vi "ADV_and_HF.vi"() -> (5 "Plug in titles":string[](array[string]), 7 "Plug in values":string[](array[string]))   [LabVIEW 2010]
uses:
  Controls/Post_Process.ctl
  Globals/Meas_global.vi
  Globals/Plug_in_data_global.vi
  <vilib>/Analysis/NI_AALBase.lvlib
panel:
  in  "Case Constant\n(See Context Help)":bool=TRUE
  out "Hot Film mean":dbl format="%.2f"
  out "ADV mean":dbl format="%.2f"
  in  "Approx period":dbl=38.0 format="%.2f"
  in  "End chop":i32
  in  "Start chop":i32
  out "Auto End Chop":i32
  out "Product":dbl[][](graph)
  out "Hot Film":dbl[][](graph)
  out "ADV":dbl[][](graph)
  out "Hot Film Auto correlation":cluster{dbl, dbl, dbl[]}(graph)
  out "ADV Auto correlation":cluster{dbl, dbl, dbl[]}[](graph)
  out "Correlation Coefficient":T1(graph)
  out "Clipped length":i32
  out "Auto Start Chop":i32
  out "V components":cluster{dbl[], dbl[]}[](graph)
  out "U components":cluster{dbl[], dbl[]}[](graph)
  # "End chop"
  # "End chop"
  # "Amount Hot Film leads ADV"
  # "End chop"
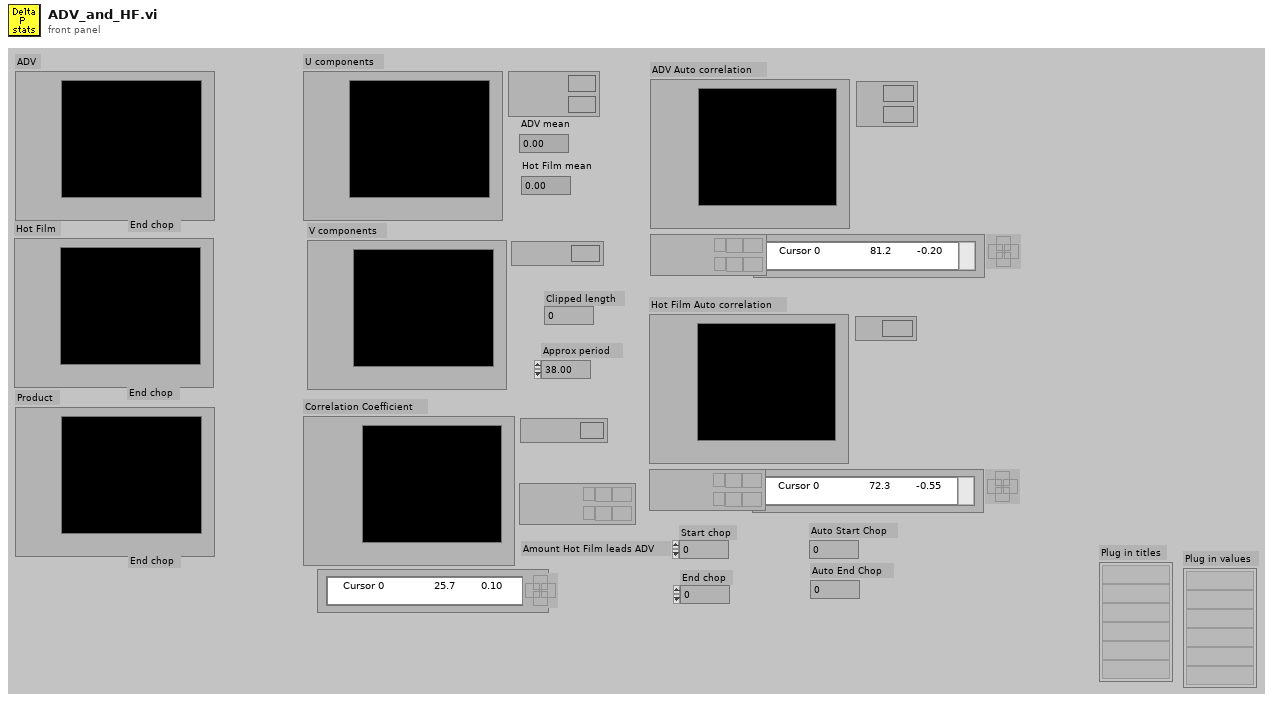
[diagram p1: front panel]
types:
  T1 = cluster{"Time":dbl[], "Correlation Coefficient":dbl[]}
  T2 = typedef "Post_Process.ctl" = enum16{"Take New Data", "Post Process Raw Data File"}
  T3 = typedef "Analysis_info_cluster.ctl" = cluster{"Colour":u32, "Inst type":T4, "Inst name":string, "Symbol":string, "Code name":string, "Extra Info":string, "Inst Array":T5, "Index":i32, "Voltage Index":i32, "Extra Titles":string[], "Extra Values":string[]}
  T4 = typedef "Inst_type.ctl" = enum16{"Propeller anemometer", "Raw voltage", "Pressure Transducer", "Pitot-static tube", "Preston tube", "Hot wire", "Cross wire 1", "Cross wire 2", "Generic Linear", "Generic Polynomial", "Generic BackPoly", "Fast FID", "Thermocouple", "Cold wire", "Pulsed Wire", "LDA Vel", "LDA Tran time", "LDA Arr time"}
  T5 = typedef "Instrument_Array.ctl" = enum16{"PWA", "LDA", "Analogue"}
  T6 = cluster{"Name":string, "X":dbl, "Y":dbl, "Z":dbl}[]
  T7 = cluster{"Name":string, "X":dbl, "Y":dbl, "Z":dbl}
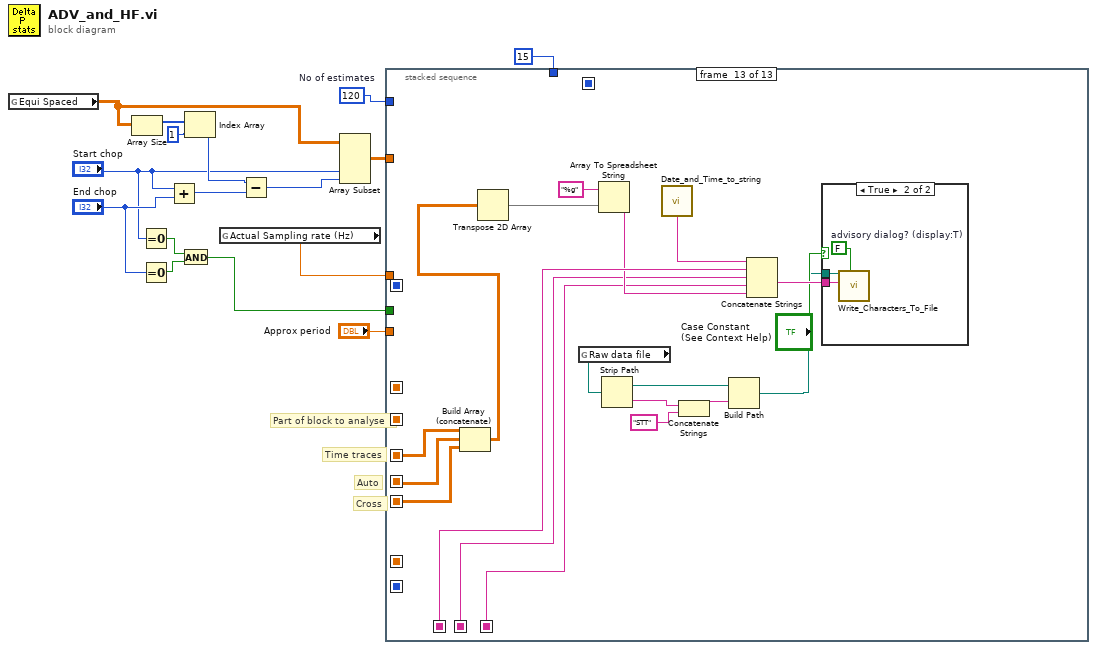
[diagram p0: block diagram]
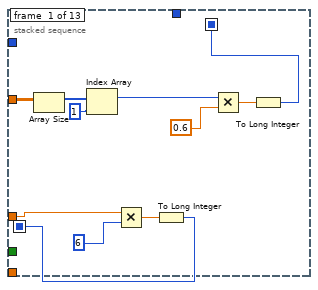
[diagram p2: hidden frame]
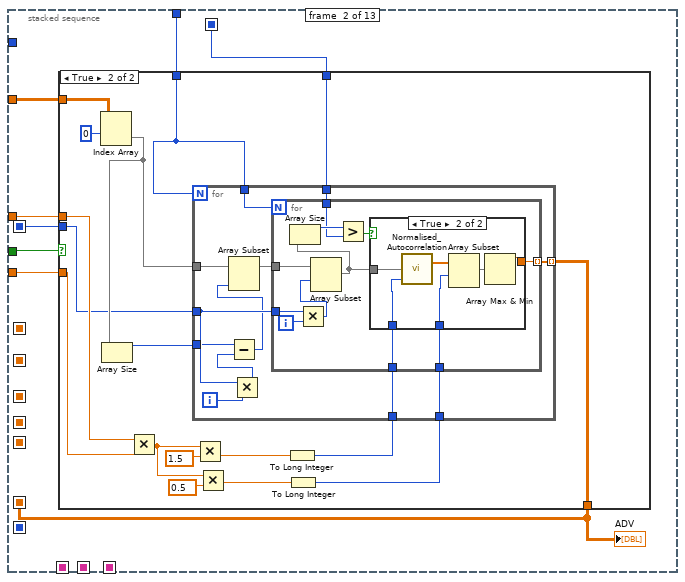
[diagram p3: hidden frame]
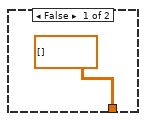
[diagram p4: hidden frame]
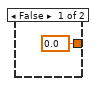
[diagram p5: hidden frame]
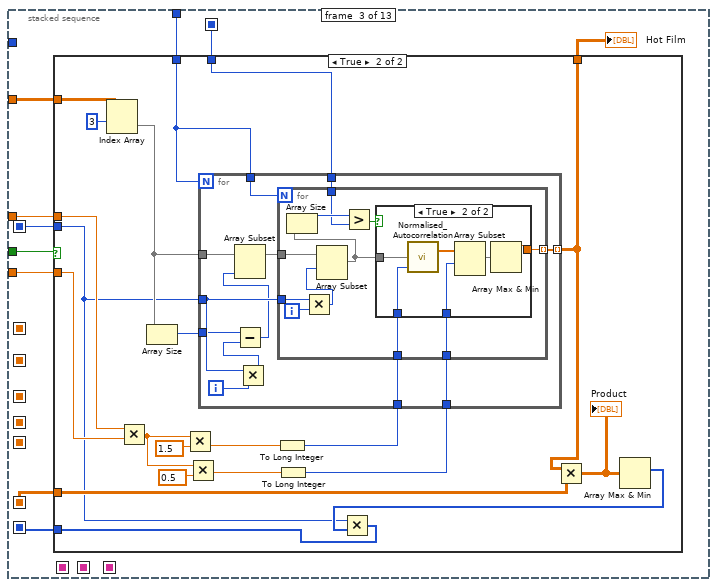
[diagram p6: hidden frame]
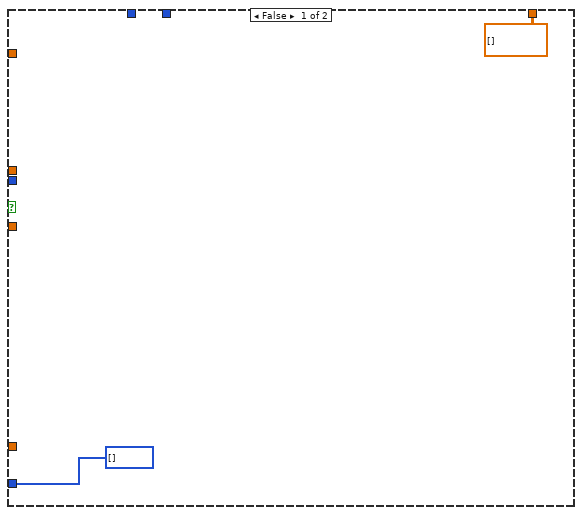
[diagram p7: hidden frame]
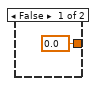
[diagram p8: hidden frame]
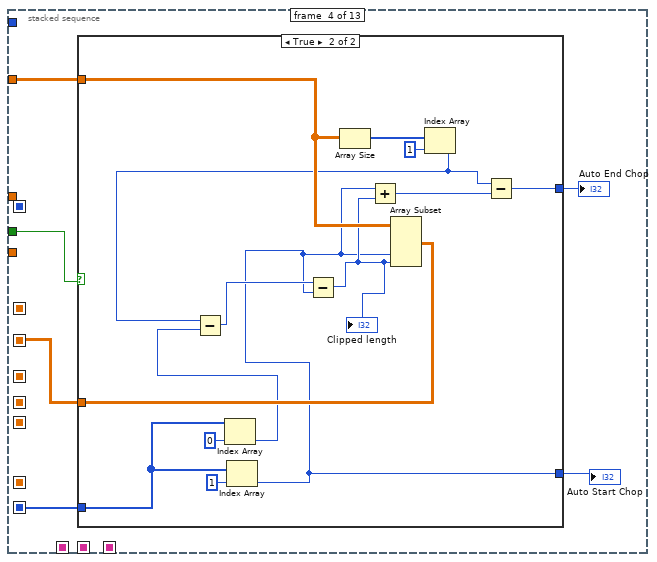
[diagram p9: hidden frame]
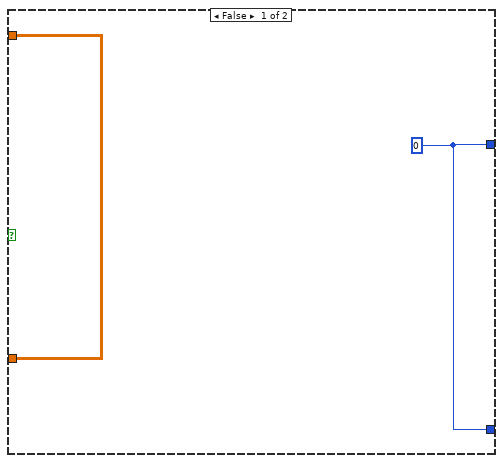
[diagram p10: hidden frame]
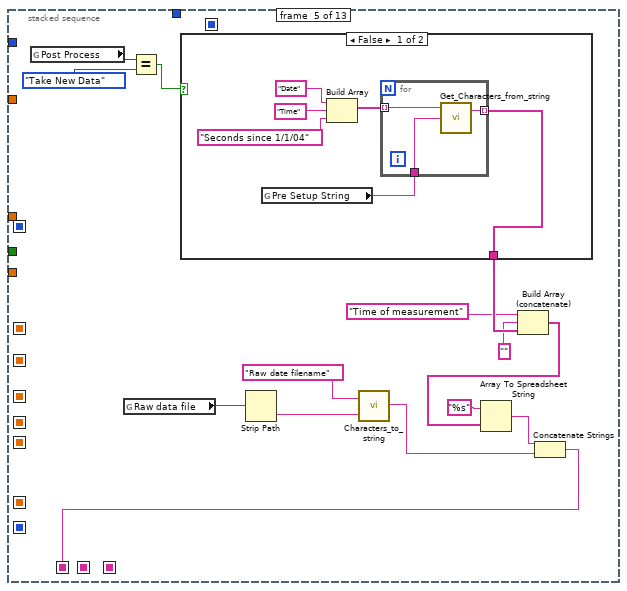
[diagram p11: hidden frame]
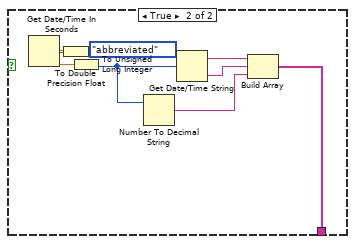
[diagram p12: hidden frame]
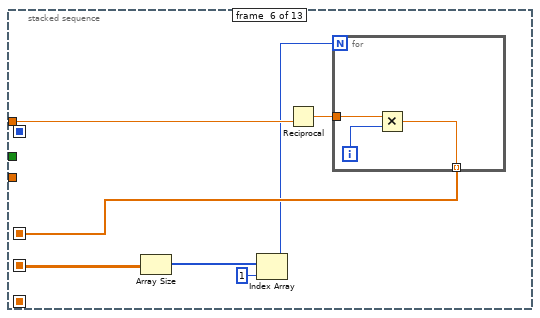
[diagram p13: hidden frame]
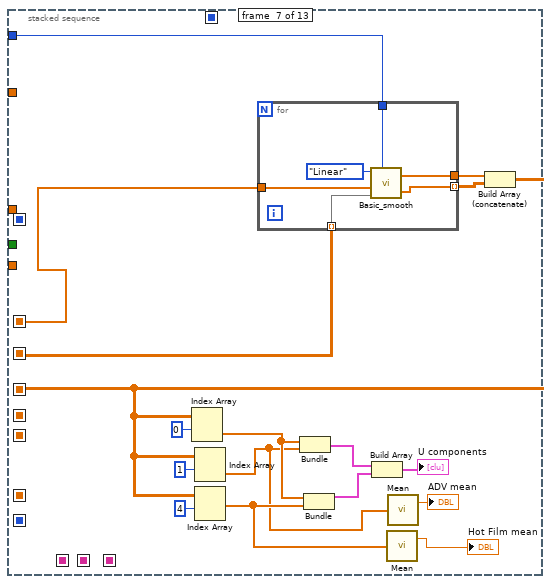
[diagram p14: hidden frame]
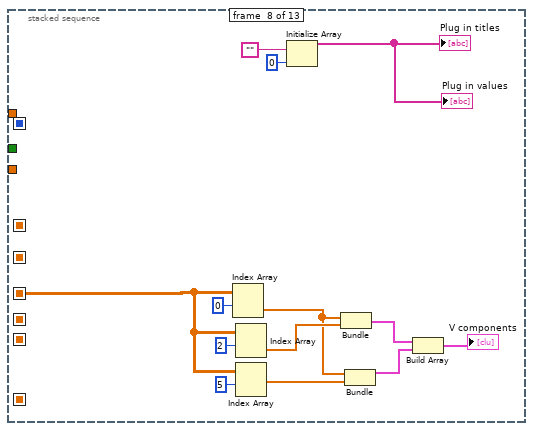
[diagram p15: hidden frame]
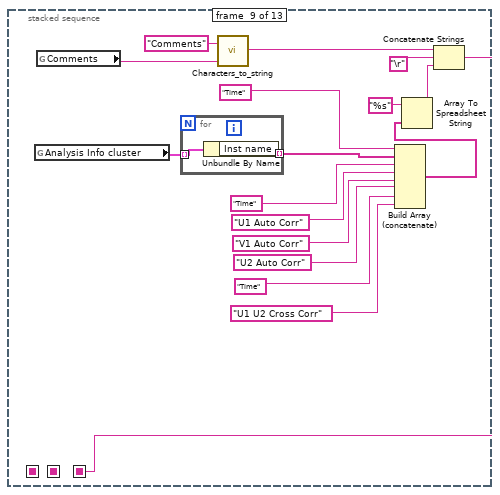
[diagram p16: hidden frame]
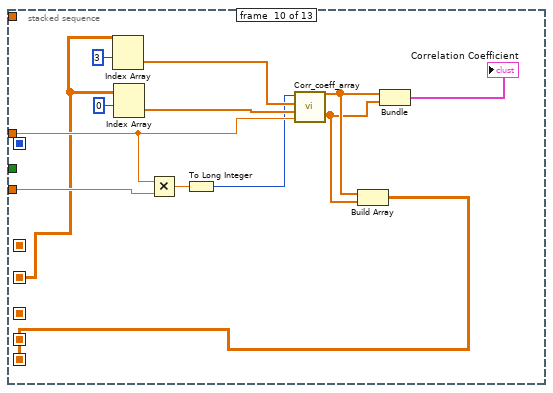
[diagram p17: hidden frame]
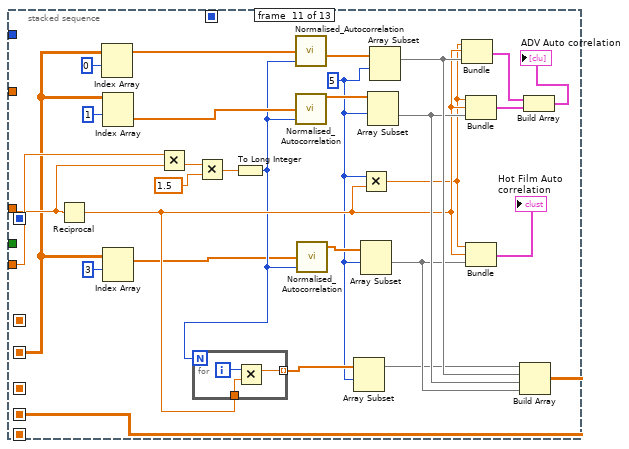
[diagram p18: hidden frame]
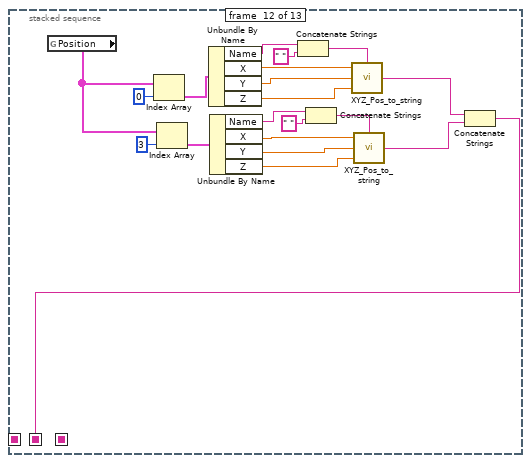
[diagram p19: hidden frame]
diagram:
  w16 = 120  # No of estimates
  # "Cross"
  # "Auto"
  # "Part of block to analyse"
  # "Time traces"
  n1 = global read "Plug_in_data_global.vi" "Equi Spaced"() -> (w7:dbl[][])
  n2 = Array Size(array=w7) -> (size(s)=w13:i32[])
  n3 = Equal To 0?(x="Start chop") -> (x = 0?=w3:bool)
  n4 = Equal To 0?(x="End chop") -> (x = 0?=w4:bool)
  n5 = Add(x="Start chop", y="End chop") -> (x+y=w11:i32)
  n6 = And(x=w3, y=w4) -> (x .and. y?=w2:bool)
  n7 = Index Array(array=w13, index=1) -> (element=w12:i32)
  n8 = global read "Meas_global.vi" "Actual Sampling rate (Hz)"() -> (w1:dbl)
  n9 = Subtract(x=w12, y=w11) -> (x-y=w10:i32)
  n10 = Array Subset(array=w7, index (col)="Start chop", length (col)=w10) -> (w15:dbl[][])  [unwired: 2 in]
  n11 = stacked-sequence {
    seq-local: [_ _ _ _ _ _ _ _ w258 _ _ _ _] -> [_ _ _ _ _ _ _ _ _ _ _ _ w337]
    seq-local: [_ _ _ _ _ w205 _ _ _ _ _ _ _] -> [_ _ _ _ _ _ w226 _ _ _ _ _ _]
    seq-local: [_ _ _ _ _ _ w218 _ _ _ _ _ _] -> [_ _ _ _ _ _ _ w234 _ _ _ _ w343]
    seq-local: [_ _ _ _ w175 _ _ _ _ _ _ _ _] -> [_ _ _ _ _ _ _ _ _ _ _ _ w347]
    seq-local: [_ _ _ w152 _ _ _ _ _ _ _ _ _] -> [_ _ _ _ _ w201 w222 _ _ w266 w282 _ _]
    seq-local: [_ _ _ _ _ _ _ _ _ _ w298 _ _] -> [_ _ _ _ _ _ _ _ _ _ _ _ w342]
    seq-local: [_ _ _ _ _ _ _ _ _ w271 _ _ _] -> [_ _ _ _ _ _ _ _ _ _ _ _ w341]
    seq-local: [_ w28 _ _ _ _ _ _ _ _ _ _ _] -> [_ _ w92 _ _ _ _ _ _ _ _ _ _]
    seq-local: [_ _ w91 _ _ _ _ _ _ _ _ _ _] -> [_ _ _ w150 _ _ _ _ _ _ _ _ _]
    seq-local: [_ _ _ _ _ _ _ _ _ _ _ w315 _] -> [_ _ _ _ _ _ _ _ _ _ _ _ w336]
    seq-local: [w18 _ _ _ _ _ _ _ _ _ _ _ _] -> [_ w34 w90 _ _ _ _ _ _ _ _ _ _]
    seq-local: [w17 _ _ _ _ _ _ _ _ _ _ _ _] -> [_ w30 w86 _ _ _ _ _ _ _ _ _ _]
    tunnel: w1 -> [w20 w32 w88 _ _ w204 _ _ _ w268 w296 _ _]
    tunnel: w16 -> [_ _ _ _ _ _ w223 _ _ _ _ _ _]
    tunnel: w15 -> [w21 w35 w93 w151 _ _ _ _ _ _ _ _ _]
    tunnel: "Approx period" -> [_ w33 w89 _ _ _ _ _ _ w269 w297 _ _]
    tunnel: 15 -> [_ w31 w87 _ _ _ _ _ _ _ _ _ _]
    tunnel: w2 -> [_ w29 w85 w149 _ _ _ _ _ _ _ _ _]
    frame #0 {
      n12 = Array Size(array=w21) -> (size(s)=w23:i32[])
      n13 = Index Array(array=w23, index=1) -> (element=w19:i32)
      n14 = Multiply(x=w20, y=6) -> (x*y=w26:dbl)
      n15 = To Long Integer(number=w26) -> (32bit integer=w17:i32)
      n16 = Multiply(x=w19, y=0.6) -> (x*y=w25:dbl)
      n17 = To Long Integer(number=w25) -> (32bit integer=w18:i32)
    }
    frame #1 {
      n18 = case shown="True" w29 {
        tunnel: w35 -> [_ w52]
        tunnel: [dbl[][] [] w49] -> w28
        tunnel: w34 -> [_ w48]
        tunnel: w33 -> [_ w40]
        tunnel: w32 -> [_ w39]
        tunnel: w31 -> [_ w38]
        tunnel: w30 -> [_ w37]
        frame False {
        }
        frame True {
          n19 = Index Array(array=w52, index (row)=0) -> (element=w51:dbl[])  [unwired: 1 in]
          n20 = Array Size(array=w51) -> (size(s)=w50:i32)
          n21 = Multiply(x=w39, y=w40) -> (x*y=w44:dbl)
          n22 = Multiply(x=w44, y=1.5) -> (x*y=w46:dbl)
          n23 = Multiply(x=w44, y=0.5) -> (x*y=w43:dbl)
          n24 = To Long Integer(number=w46) -> (32bit integer=w42:i32)
          n25 = To Long Integer(number=w43) -> (32bit integer=w41:i32)
          n26 = for {
            N: w38 -> [_]
            tunnel: w37 -> [w63]
            tunnel: w51 -> [w59]
            tunnel: w38 -> [w65]
            tunnel: w50 -> [w62]
            tunnel: [w57] -> w49 mode=indexing
            tunnel: w48 -> [w56]
            tunnel: w42 -> [w55]
            tunnel: w41 -> [w54]
            i -> [w64]
            n27 = Multiply(x=w63, y=w64) -> (x*y=w61:i32)
            n28 = Subtract(x=w62, y=w61) -> (x-y=w60:i32)
            n29 = Array Subset(array=w59, length=w60) -> (w58:dbl[])  [unwired: 1 in]
            n30 = for {
              N: w65 -> [_]
              tunnel: w63 -> [w74]
              tunnel: w58 -> [w73]
              tunnel: [w72] -> w57 mode=indexing
              tunnel: w56 -> [w68]
              tunnel: w55 -> [w67]
              tunnel: w54 -> [w66]
              i -> [w76]
              n31 = Multiply(x=w74, y=w76) -> (x*y=w75:i32)
              n32 = Array Subset(array=w73, index=w75) -> (w71:dbl[])  [unwired: 1 in]
              n33 = Array Size(array=w71) -> (size(s)=w69:i32)
              n34 = Greater?(x=w69, y=w68) -> (0:w70:bool)
              n35 = case shown="True" w70 {
                tunnel: [0.0 w83] -> w72
                tunnel: w71 -> [_ w80]
                tunnel: w67 -> [_ w79]
                tunnel: w66 -> [_ w78]
                frame False {
                }
                frame True {
                  n36 = call "Normalised_Autocorrelation.vi"("Autocorrelation length"=w79, "Array"=w80) -> ("Normalised Auto corr"=w82:dbl[])  [unwired: 1 in]
                  n37 = Array Subset(array=w82, index=w78) -> (w81:dbl[])  [unwired: 1 in]
                  n38 = Array Max & Min(array=w81) -> (max value=w83:dbl)  [unwired: 3 out]
                }
              }
            }
          }
        }
      }
      "ADV" <- w28
    }
    frame #2 {
      n39 = case shown="True" w85 {
        tunnel: w93 -> [_ w115]
        tunnel: w92 -> [_ w114]
        tunnel: [i32[] [] w111] -> w91
        tunnel: w90 -> [_ w108]
        tunnel: w89 -> [_ w105]
        tunnel: w88 -> [_ w104]
        tunnel: w87 -> [_ w98]
        tunnel: w86 -> [_ w97]
        tunnel: [dbl[][] [] w96] -> w84
        frame False {
        }
        frame True {
          n40 = Index Array(array=w115, index (row)=3) -> (element=w110:dbl[])  [unwired: 1 in]
          n41 = Multiply(x=w104, y=w105) -> (x*y=w101:dbl)
          n42 = Array Size(array=w110) -> (size(s)=w109:i32)
          n43 = Multiply(x=w101, y=1.5) -> (x*y=w106:dbl)
          n44 = Multiply(x=w101, y=0.5) -> (x*y=w100:dbl)
          n45 = To Long Integer(number=w106) -> (32bit integer=w103:i32)
          n46 = To Long Integer(number=w100) -> (32bit integer=w99:i32)
          n47 = for {
            N: w98 -> [_]
            tunnel: w97 -> [w126]
            tunnel: w110 -> [w122]
            tunnel: w98 -> [w128]
            tunnel: w109 -> [w125]
            tunnel: [w120] -> w96 mode=indexing
            tunnel: w108 -> [w119]
            tunnel: w103 -> [w118]
            tunnel: w99 -> [w117]
            i -> [w127]
            n48 = Multiply(x=w126, y=w127) -> (x*y=w124:i32)
            n49 = Subtract(x=w125, y=w124) -> (x-y=w123:i32)
            n50 = Array Subset(array=w122, length=w123) -> (w121:dbl[])  [unwired: 1 in]
            n51 = for {
              N: w128 -> [_]
              tunnel: w126 -> [w137]
              tunnel: w121 -> [w136]
              tunnel: [w135] -> w120 mode=indexing
              tunnel: w119 -> [w131]
              tunnel: w118 -> [w130]
              tunnel: w117 -> [w129]
              i -> [w139]
              n52 = Multiply(x=w137, y=w139) -> (x*y=w138:i32)
              n53 = Array Subset(array=w136, index=w138) -> (w134:dbl[])  [unwired: 1 in]
              n54 = Array Size(array=w134) -> (size(s)=w132:i32)
              n55 = Greater?(x=w132, y=w131) -> (0:w133:bool)
              n56 = case shown="True" w133 {
                tunnel: [0.0 w146] -> w135
                tunnel: w134 -> [_ w143]
                tunnel: w130 -> [_ w142]
                tunnel: w129 -> [_ w141]
                frame False {
                }
                frame True {
                  n57 = call "Normalised_Autocorrelation.vi"("Autocorrelation length"=w142, "Array"=w143) -> ("Normalised Auto corr"=w145:dbl[])  [unwired: 1 in]
                  n58 = Array Subset(array=w145, index=w141) -> (w144:dbl[])  [unwired: 1 in]
                  n59 = Array Max & Min(array=w144) -> (max value=w146:dbl)  [unwired: 3 out]
                }
              }
            }
          }
          n60 = Multiply(x=w96, y=w114) -> (x*y=w113:dbl[][])
          "Product" <- w113
          n61 = Array Max & Min(array=w113) -> (max index (indices)=w112:i32[])  [unwired: 3 out]
          n62 = Multiply(x=w97, y=w112) -> (x*y=w111:i32[])
        }
      }
      "Hot Film" <- w84
    }
    frame #3 {
      n63 = case shown="True" w149 {
        tunnel: [w154 w168] -> w152
        tunnel: w151 -> [w154 w167]
        tunnel: w150 -> [_ w161]
        tunnel: [w153 w156] -> w148
        tunnel: [w153 w155] -> w147
        frame False {
          w153 = 0
        }
        frame True {
          n64 = Index Array(array=w161, index=0) -> (element=w163:i32)
          n65 = Index Array(array=w161, index=1) -> (element=w155:i32)
          n66 = Array Size(array=w167) -> (size(s)=w165:i32[])
          n67 = Index Array(array=w165, index=1) -> (element=w158:i32)
          n68 = Subtract(x=w158, y=w163) -> (x-y=w160:i32)
          n69 = Subtract(x=w160, y=w155) -> (x-y=w159:i32)
          "Clipped length" <- w159
          n70 = Add(x=w155, y=w159) -> (x+y=w157:i32)
          n71 = Array Subset(array=w167, index (col)=w155, length (col)=w159) -> (w168:dbl[][])  [unwired: 2 in]
          n72 = Subtract(x=w158, y=w157) -> (x-y=w156:i32)
        }
      }
      "Auto End Chop" <- w148
      "Auto Start Chop" <- w147
    }
    frame #4 {
      n73 = global read "Meas_global.vi" "Post Process"() -> (w181:T2)
      n74 = global read "Meas_global.vi" "Raw data file"() -> (w170:path)
      n75 = Equal?(x=w181, y=Post_Process."Take New Data" ("Post Process")) -> (x = y?=w180:bool)
      n76 = case shown="False" w180 {
        tunnel: [w183 w193] -> w174
        frame False {
          n77 = global read "Meas_global.vi" "Pre Setup String"() -> (w184:string)
          n78 = Build Array("Date", "Time", "Seconds since 1/1/04") -> (w185:string[])
          n79 = for {
            tunnel: w185 -> [w191] mode=indexing
            tunnel: w184 -> [w190]
            tunnel: [w189] -> w183 mode=indexing
            n80 = call "Get_Characters_from_string.vi"("Input string"=w190, "Variable name"=w191) -> ("Value"=w189:string)  [unwired: 1 in, 1 out]
          }
        }
        frame True {
          n81 = Get Date/Time In Seconds() -> (seconds since 1Jan1904=w192:timestamp)
          n82 = To Double Precision Float(number=w192) -> (double precision float=w196:dbl)
          n83 = To Unsigned Long Integer(number=w196) -> (unsigned 32bit integer=w195:u32)
          n84 = Number To Decimal String(number=w195) -> (decimal integer string=w194:string)  [unwired: 1 in]
          n85 = Get Date/Time String(date format (0)=enum16{"short", "long", "abbreviated"}."abbreviated", seconds (now)=w195) -> (date string=w198:string, time string=w197:string)  [unwired: 1 in]
          n86 = Build Array(w198, w197, w194) -> (w193:string[])
        }
      }
      n87 = Strip Path(path=w170) -> (name=w169:string)  [unwired: 1 out]
      n88 = call "Characters_to_string.vi"("Characters to write"=w169, "Label for characters"="Raw date filename") -> ("Output string"=w176:string)
      n89 = Build Array (concatenate)("Time of measurement", "" ("Value"), w174) -> (w171:string[])
      n90 = Array To Spreadsheet String(array=w171, 3:"%s" ("format string")) -> (spreadsheet string=w177:string)  [unwired: 1 in]
      n91 = Concatenate Strings(w177, w176) -> (w175:string)
    }
    frame #5 {
      n92 = Array Size(array=w201) -> (size(s)=w202:i32[])
      n93 = Index Array(array=w202, index=1) -> (element=w200:i32)
      n94 = Reciprocal(x=w204) -> (1/x=w206:dbl)
      n95 = for {
        N: w200 -> [_]
        tunnel: w206 -> [w209]
        tunnel: [w207] -> w205 mode=indexing
        i -> [w208]
        n96 = Multiply(x=w209, y=w208) -> (x*y=w207:dbl)
      }
    }
    frame #6 {
      n97 = for {
        tunnel: w226 -> [w231]
        tunnel: w222 -> [w230] mode=indexing
        tunnel: [w229] -> w225
        tunnel: [w228] -> w224 mode=indexing
        tunnel: w223 -> [w227]
        n98 = call "Basic_smooth.vi"("Smoothing"=enum16{"Linear", "Logarithmic"}."Linear", "X array in"=w231, "Y array in"=w230, "No of estimates output"=w227) -> ("X array Out"=w229:dbl[], "Y array Out"=w228:dbl[])  [unwired: 1 in]
      }
      n99 = Build Array (concatenate)(w225, w224) -> (w218:dbl[][])
      n100 = Index Array(array=w218, index (row)=0) -> (element=w217:dbl[])  [unwired: 1 in]
      n101 = Index Array(array=w218, index (row)=1) -> (element=w212:dbl[])  [unwired: 1 in]
      n102 = Index Array(array=w218, index (row)=4) -> (element=w213:dbl[])  [unwired: 1 in]
      n103 = Bundle(w217, w212) -> (w216:cluster{dbl[], dbl[]})  [unwired: 1 in]
      n104 = Bundle(w217, w213) -> (w215:cluster{dbl[], dbl[]})  [unwired: 1 in]
      n105 = Build Array(w216, w215) -> (→"U components":cluster{dbl[], dbl[]}[])
      n106 = call <vilib>:"Mean.vi"("X"=w213) -> ("mean"=→"Hot Film mean":dbl)  [unwired: 1 out]
      n107 = call <vilib>:"Mean.vi"("X"=w212) -> ("mean"=→"ADV mean":dbl)  [unwired: 1 out]
    }
    frame #7 {
      n108 = Index Array(array=w234, index (row)=0) -> (element=w238:dbl[])  [unwired: 1 in]
      n109 = Index Array(array=w234, index (row)=2) -> (element=w240:dbl[])  [unwired: 1 in]
      n110 = Index Array(array=w234, index (row)=5) -> (element=w237:dbl[])  [unwired: 1 in]
      n111 = Initialize Array("", 0) -> (→"Plug in titles" →"Plug in values":string[])
      n112 = Bundle(w238, w240) -> (w236:cluster{dbl[], dbl[]})  [unwired: 1 in]
      n113 = Bundle(w238, w237) -> (w235:cluster{dbl[], dbl[]})  [unwired: 1 in]
      n114 = Build Array(w236, w235) -> (→"V components":cluster{dbl[], dbl[]}[])
    }
    frame #8 {
      n115 = global read "Meas_global.vi" "Analysis Info cluster"() -> (w257:T3[])
      n116 = global read "Meas_global.vi" "Comments"() -> (w262:string)
      n117 = for {
        tunnel: w257 -> [w264] mode=indexing
        tunnel: [w263] -> w248 mode=indexing
        n118 = Unbundle By Name(w264) -> ("Inst name"=w263:string)
      }
      n119 = call "Characters_to_string.vi"("Characters to write"=w262, "Label for characters"="Comments") -> ("Output string"=w260:string)
      n120 = Build Array (concatenate)("Time", w248, "Time", "U1 Auto Corr", "V1 Auto Corr", "U2 Auto Corr", "Time", "U1 U2 Cross Corr") -> (w251:string[])
      n121 = Array To Spreadsheet String(array=w251, 3:"%s" ("format string")) -> (spreadsheet string=w250:string)  [unwired: 1 in]
      n122 = Concatenate Strings(w260, "\r", w250) -> (w258:string)
    }
    frame #9 {
      n123 = Index Array(array=w266, index (row)=3) -> (element=w277:dbl[])  [unwired: 1 in]
      n124 = Index Array(array=w266, index (row)=0) -> (element=w276:dbl[])  [unwired: 1 in]
      n125 = Multiply(x=w268, y=w269) -> (x*y=w267:dbl)
      n126 = To Long Integer(number=w267) -> (32bit integer=w265:i32)
      n127 = call "Corr_coeff_array.vi"("Sampling frequency"=w268, "U2"=w276, "U1"=w277, "Slippage range"=w265) -> ("Correlation Coefficient"=w272:dbl[], "Time"=w273:dbl[])
      n128 = Build Array(w273, w272) -> (w271:dbl[][])
      n129 = Bundle("Time"=w273, "Correlation Coefficient"=w272) -> (→"Correlation Coefficient":T1)  [unwired: 1 in]
    }
    frame #10 {
      w281 = 5
      n130 = Reciprocal(x=w296) -> (1/x=w284:dbl)
      n131 = Index Array(array=w282, index (row)=0) -> (element=w302:dbl[])  [unwired: 1 in]
      n132 = Index Array(array=w282, index (row)=1) -> (element=w306:dbl[])  [unwired: 1 in]
      n133 = Index Array(array=w282, index (row)=3) -> (element=w278:dbl[])  [unwired: 1 in]
      n134 = Multiply(x=w297, y=w296) -> (x*y=w295:dbl)
      n135 = Multiply(x=w295, y=1.5) -> (x*y=w293:dbl)
      n136 = To Long Integer(number=w293) -> (32bit integer=w280:i32)
      n137 = for {
        N: w280 -> [_]
        tunnel: w284 -> [w308]
        tunnel: [w307] -> w286 mode=indexing
        i -> [w309]
        n138 = Multiply(x=w309, y=w308) -> (x*y=w307:dbl)
      }
      n139 = call "Normalised_Autocorrelation.vi"("Autocorrelation length"=w280, "Array"=w302) -> ("Normalised Auto corr"=w292:dbl[])  [unwired: 1 in]
      n140 = call "Normalised_Autocorrelation.vi"("Autocorrelation length"=w280, "Array"=w306) -> ("Normalised Auto corr"=w290:dbl[])  [unwired: 1 in]
      n141 = call "Normalised_Autocorrelation.vi"("Autocorrelation length"=w280, "Array"=w278) -> ("Normalised Auto corr"=w291:dbl[])  [unwired: 1 in]
      n142 = Array Subset(array=w286, index=w281) -> (w285:dbl[])  [unwired: 1 in]
      n143 = Multiply(x=w281, y=w284) -> (x*y=w283:dbl)
      n144 = Array Subset(array=w291, index=w281) -> (w287:dbl[])  [unwired: 1 in]
      n145 = Array Subset(array=w290, index=w281) -> (w288:dbl[])  [unwired: 1 in]
      n146 = Array Subset(array=w292, index=w281) -> (w289:dbl[])  [unwired: 1 in]
      n147 = Bundle(w283, w284, w289) -> (w300:cluster{dbl, dbl, dbl[]})  [unwired: 1 in]
      n148 = Bundle(w283, w284, w288) -> (w299:cluster{dbl, dbl, dbl[]})  [unwired: 1 in]
      n149 = Bundle(w283, w284, w287) -> (→"Hot Film Auto correlation":cluster{dbl, dbl, dbl[]})  [unwired: 1 in]
      n150 = Build Array(w285, w289, w288, w287) -> (w298:dbl[][])
      n151 = Build Array(w300, w299) -> (→"ADV Auto correlation":cluster{dbl, dbl, dbl[]}[])
    }
    frame #11 {
      n152 = global read "Meas_global.vi" "Position"() -> (w327:T6)
      n153 = Index Array(array=w327, index=0) -> (element=w326:T7)
      n154 = Index Array(array=w327, index=3) -> (element=w325:T7)
      n155 = Unbundle By Name(w326) -> ("Name"=w312:string, "X"=w323:dbl, "Y"=w322:dbl, "Z"=w321:dbl)
      n156 = Unbundle By Name(w325) -> ("Name"=w310:string, "X"=w320:dbl, "Y"=w319:dbl, "Z"=w318:dbl)
      n157 = Concatenate Strings(w312, " " ("Output string")) -> (w324:string)
      n158 = Concatenate Strings(w310, " " ("Output string")) -> (w314:string)
      n159 = call "XYZ_Pos_to_string.vi"("Position label"=w324, "Z"=w321, "Y"=w322, "X"=w323) -> ("Output string"=w317:string)
      n160 = call "XYZ_Pos_to_string.vi"("Position label"=w314, "Z"=w318, "Y"=w319, "X"=w320) -> ("Output string"=w316:string)
      n161 = Concatenate Strings(w317, w316) -> (w315:string)
    }
    frame #12 {
      n162 = Build Array (concatenate)(w343, w342, w341) -> (w339:dbl[][])
      n163 = Transpose 2D Array(2D array=w339) -> (transposed array=w348:dbl[][])
      n164 = global read "Meas_global.vi" "Raw data file"() -> (w334:path)
      n165 = Array To Spreadsheet String(array=w348, 3:"%g" ("format string")) -> (spreadsheet string=w338:string)  [unwired: 1 in]
      n166 = Strip Path(path=w334) -> (stripped path=w331:path, name=w333:string)
      n167 = call "Date_and_Time_to_string.vi"() -> ("Date and time (spreadsheet)"=w340:string)
      n168 = Concatenate Strings(w333, "STT") -> (w332:string)
      n169 = Build Path(base path=w331, name or relative path=w332) -> (appended path=w330:path)
      n170 = Concatenate Strings(w340, w347, w336, w337, w338) -> (w345:string)
      n171 = case shown="True" "Case Constant\n(See Context Help)" {
        tunnel: w345 -> [_ w351]
        tunnel: w330 -> [_ w350]
        frame False {
        }
        frame True {
          w349 = FALSE  # advisory dialog? (display:T)
          n172 = call "Write_Characters_To_File.vi"("file path (dialog if empty)"=w350, "advisory dialog? (display:T)"=w349, "character string"=w351) -> ()  [unwired: 5 in, 1 out]
        }
      }
    }
  }
